vi "Read Message Data.vi"(8 "error in (no error)":errorcluster, 11 "SECS-II Class in":refnum<class "SECS-II Class.lvclass">) -> (0 "error out":errorcluster, 1 "Empty?":bool, 2 "Message Data":T1[](array[typedef]), 3 "SECS-II Class out":refnum<class "SECS-II Class.lvclass">)   [LabVIEW 2020, in "SECS Communication.lvlib" / "SECS-II Class.lvclass"]
uses:
  SECS-II Class.lvclass
  Message Data.ctl
  Data Item Format.ctl
  Format Code.ctl
  SECS-II Class.lvclass/SECS-II Class.ctl
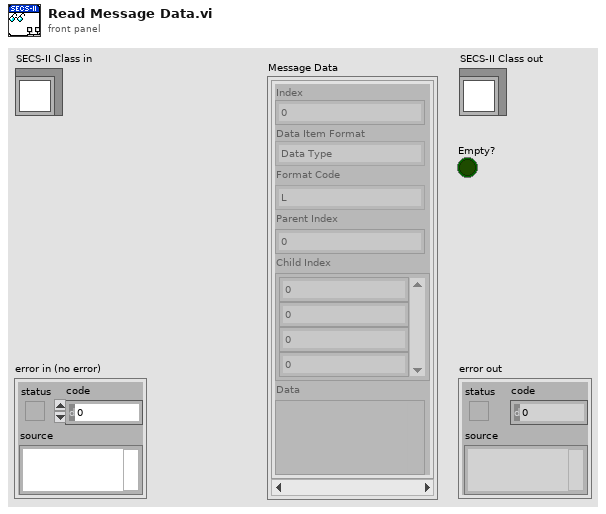
[diagram p1: front panel]
types:
  T1 = typedef "SECS Communication.lvlib/SECS-II Class.lvclass/Message Data.ctl" = cluster{"Index":i32, "Data Item Format":T2, "Format Code":T3, "Parent Index":i32, "Child Index":i32[], "Data":variant}
  T2 = typedef "SECS Communication.lvlib/SECS-II Class.lvclass/Data Item Format.ctl" = enum16{"Data Type", "Value"}
  T3 = typedef "SECS Communication.lvlib/SECS-II Class.lvclass/Format Code.ctl" = enum16{"L", "A", "B", "Boolean", "J", "I1", "I2", "I4", "I8", "U1", "U2", "U4", "U8", "F4", "F8", "Char"}
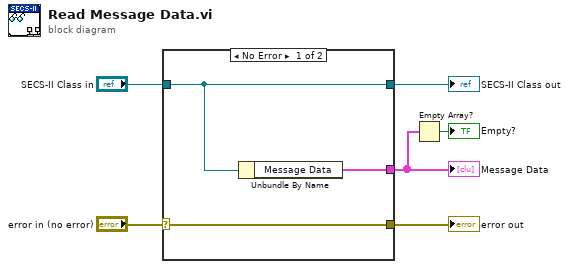
[diagram p0: block diagram]
diagram:
  n1 = case shown="No Error" "error in (no error)" {
    selector: "error in (no error)" -> [w9 w10]
    tunnel: [w9 w10] -> w5
    tunnel: [w8 w11] -> w3
    tunnel: "SECS-II Class in" -> [w8 w11]
    tunnel: [w7 _] -> w2
    frame No Error {
      n2 = Unbundle By Name(w8) -> ("Message Data"=w7:T1[])
    }
    frame Error {
    }
  }
  "error out" <- w5
  "SECS-II Class out" <- w3
  "Message Data" <- w2
  n3 = Empty Array?(array=w2) -> (empty?=→"Empty?":bool)
